vi "M05 Hydraulics.vi"(11 "NXT/EV3":T1) -> (3 "NXT/EV3 2":T1)   [LabVIEW 2016]
uses:
  <vilib>/NXT/Subs/LVHSConnector.ctl
  <vilib>/NXT/LegoClasses/BrickReference/BrickReference.lvclass
  <vilib>/NXT/Block Support/NXT_InputPort.ctl
  <vilib>/NXT/Block Support/NXT_OutputPort.ctl
  <vilib>/NXT/Dual Mode Library/Waits/Wait_Num.vi
  <vilib>/NXT/NXTIO Xnodes/NXTIONodeSubVIs/LEGOResetMotors.vi
  <vilib>/NXT/NXTIO Xnodes/NXTIONodeSubVIs/NXTMotorRunDistance.vi
  <vilib>/NXT/NXTIO Xnodes/AddressXNode/NXTIOAddress.xnode
  <vilib>/NXT/NXTIO Xnodes/NXTIOXNode/NXTIO.xnode
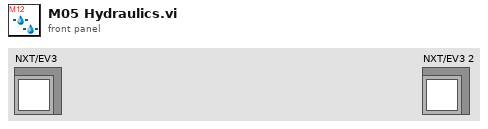
[diagram p1: front panel]
types:
  T1 = typedef "LVHSConnector.ctl" = refnum<class "BrickReference.lvclass">
  T2 = typedef "NXT_InputPort.ctl" = u32
  T3 = typedef "NXT_OutputPort.ctl" = u8
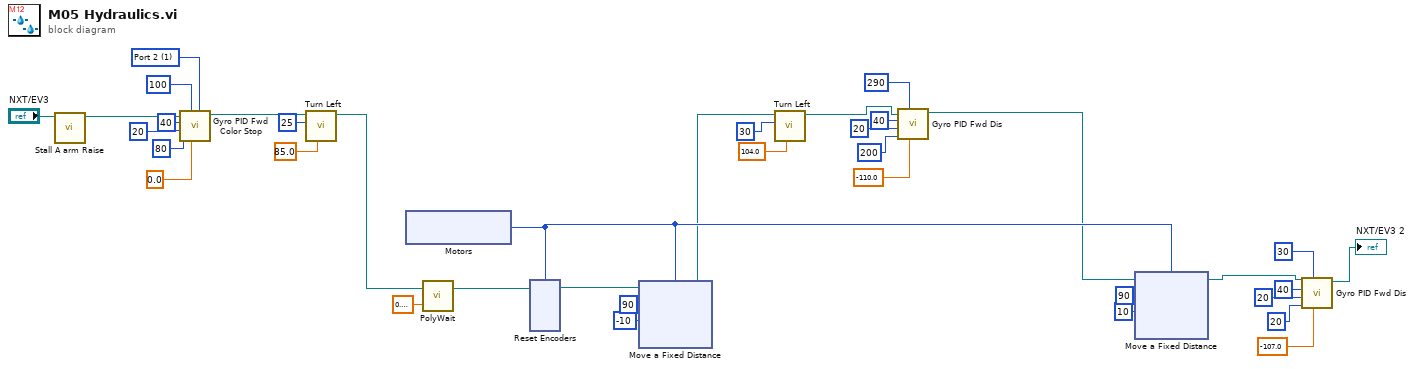
[diagram p0: block diagram]
diagram:
  w23 = T2 1 items=["Port 1", "Port 2", "Port 3", "Port 4"] ("Port")
  n1 = call "Stall A arm Raise.vi"("NXT/EV3"="NXT/EV3") -> ("NXT/EV3"=w24:T1)  [unwired: 10 in]
  n2 = call "Gyro PID Fwd Color Stop.vi"("Port"=w23, "Target angle"=sgl 0.0, "Threshold to Color"=100, "Threshold to slow"=80, "Min. speed"=20, "Max. speed"=40, "EV3 in"=w24) -> ("EV3 out"=w17:T1)  [unwired: 4 in]
  n3 = call "Turn Left.vi"("Turning angle"=sgl 85.0, "Motor B (right)"=i8 25, "EV3 in"=w17) -> ("EV3 out"=w16:T1)  [unwired: 8 in]
  n4 = xnode "Motors"() -> ("Motor"=w13:T3)
  n5 = call-poly <vilib>:"PolyWait.vi"("Time (1 sec)"=sgl 0.3, "NXT/EV3"=w16) -> ("NXT/EV3"=w35:T1)  [unwired: 2 in]
  n6 = xnode "Reset Encoders"("Motors"=w13, "NXT/EV3"=w35) -> ("NXT/EV3"=w34:T1)
  n7 = xnode "Move a Fixed Distance"("Speed 1"=i8 -10, "Distance 1"=90, "Motors"=w13, "NXT/EV3"=w34) -> ("NXT/EV3"=w9:T1)
  n8 = call "Turn Left.vi"("Turning angle"=sgl 104.0, "Motor B (right)"=i8 30, "EV3 in"=w9) -> ("EV3 out"=w10:T1)  [unwired: 8 in]
  n9 = call "Gyro PID Fwd Dis.vi"("Target angle"=sgl -110.0, "Threshold to stop"=290, "Threshold to slow"=200, "Min. speed"=20, "Max. speed"=40, "EV3 in"=w10) -> ("EV3 out"=w8:T1)  [unwired: 5 in]
  n10 = xnode "Move a Fixed Distance"("Speed 1"=i8 10, "Distance 1"=90, "Motors"=w13, "NXT/EV3"=w8) -> ("NXT/EV3"=w2:T1)
  n11 = call "Gyro PID Fwd Dis.vi"("Target angle"=sgl -107.0, "Threshold to stop"=30, "Threshold to slow"=20, "Min. speed"=20, "Max. speed"=40, "EV3 in"=w2) -> ("EV3 out"=→"NXT/EV3 2":T1)  [unwired: 5 in]
